vi "Get RPM.vi"(8 "error in (no error)":errorcluster, 11 "Ismatech 3 Channel Settings In":T1={"VISA resource name"="", "Pump Number"=1, "Channel Number"=0, "Simulated?"=TRUE, "Reverse?"=FALSE} {"Channel Number" min=0 max=3; "Pump Number" min=1 max=9}) -> (0 "error out":errorcluster, 2 "RPM":dbl, 3 "Ismatech 3 Channel Settings Out":T1={"VISA resource name"="", "Pump Number"=1, "Channel Number"=0, "Simulated?"=TRUE, "Reverse?"=FALSE} {"Channel Number" min=0 max=3; "Pump Number" min=1 max=9})   [LabVIEW 2018, in "Ismatec 4308.lvlib"]
uses:
  Ismatec 4308.lvlib
  Ismatec 4083.ctl
  support/Support Library.lvlib
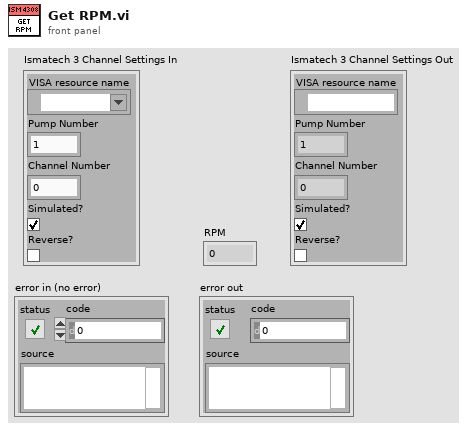
[diagram p1: front panel]
types:
  T1 = typedef "Ismatec 4308.lvlib/Ismatec 4083.ctl" = cluster{"VISA resource name":refnum<visa-resource-name>, "Pump Number":i16, "Channel Number":i16, "Simulated?":bool, "Reverse?":bool}
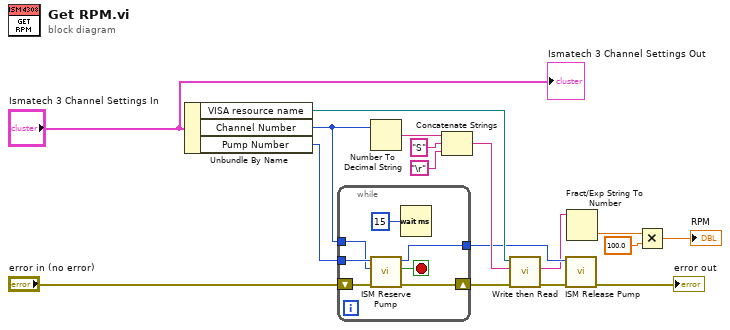
[diagram p0: block diagram]
diagram:
  n1 = Unbundle By Name("Ismatech 3 Channel Settings In") -> ("VISA resource name"=w11:refnum<visa-resource-name>, "Channel Number"=w7:i16, "Pump Number"=w8:i16)
  n2 = while {
    tunnel: w8 -> [w22]
    tunnel: w7 -> [w21]
    shift-right: [w23] -> w4
    shift-left: "error in (no error)" -> [w24]
    tunnel: [w18] -> w5
    stop <- w20 stop-if-true
    n3 = call "ISM Reserve Pump.vi"("error in (no error)"=w24, "ISM Channel # In"=w21, "ISM Pump # In"=w22) -> ("error out"=w23:errorcluster, "Loop Completed"=w20:bool, "ISM Pump # Out"=w18:i32)  [unwired: 6 in]
    n4 = Wait (ms)(milliseconds to wait=u32 15) -> ()  [unwired: 1 out]
  }
  n5 = Number To Decimal String(number=w7) -> (decimal integer string=w14:string)  [unwired: 1 in]
  n6 = Concatenate Strings(w14, "S", "\r") -> (w10:string)
  n7 = call "Write then Read.vi"("error in"=w4, "write buffer"=w10, "VISA resource name in"=w11) -> ("error out"=w9:errorcluster, "read buffer"=w2:string)  [unwired: 5 in, 2 out]
  n8 = call "ISM Release Pump.vi"("error in (no error)"=w9, "Pump Number In"=w5) -> ("error out"=→"error out":errorcluster)  [unwired: 8 in, 1 out]
  n9 = Fract/Exp String To Number(string=w2) -> (number=w3:dbl)  [unwired: 3 in, 1 out]
  n10 = Multiply(x=w3, y=100.0) -> (x*y=→"RPM":dbl)
  "Ismatech 3 Channel Settings Out" <- "Ismatech 3 Channel Settings In"
